vi "gmail 8.2.vi"(0 "Recipient's Email Address Address":string, 1 "Subject":string, 2 "Sender's Email Address (eg: jsmith77@gmail.com)":string, 3 "Recipient's Name":string, 4 "CC (Carbon Copy Recipient - Optional)":string, 5 "Body":string="It works!", 8 "Attachment - Optional":path) -> ()   [LabVIEW 2010]
panel:
  in  "Port":i32=587
  in  "Enable SSL":bool=TRUE
  in  "GMAIL Account Password":string="Tigger88"
  in  "GMAIL Account User ID (eg: jsmity77)":string="logan.t.meyer@gmail.com"
  in  "Outgoing Mail Server (SMTP)":string="smtp.gmail.com"
  in  "Sender's Name":string="Logan Meyer"
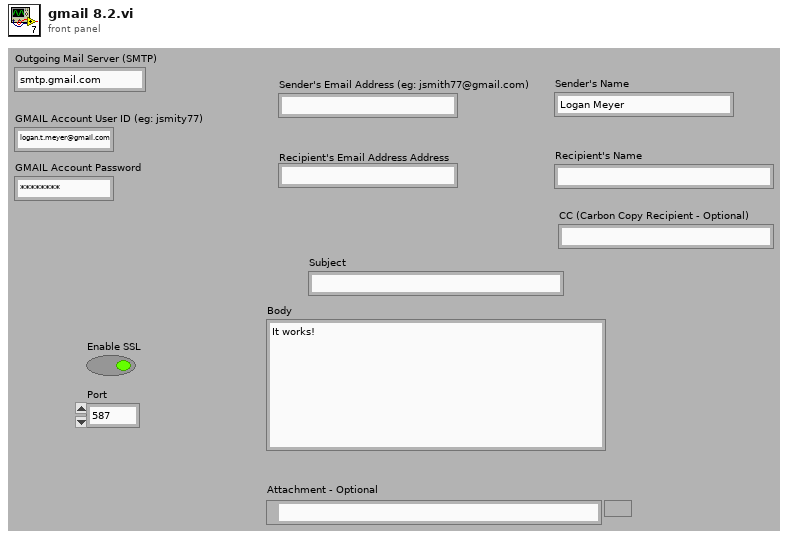
[diagram p1: front panel]
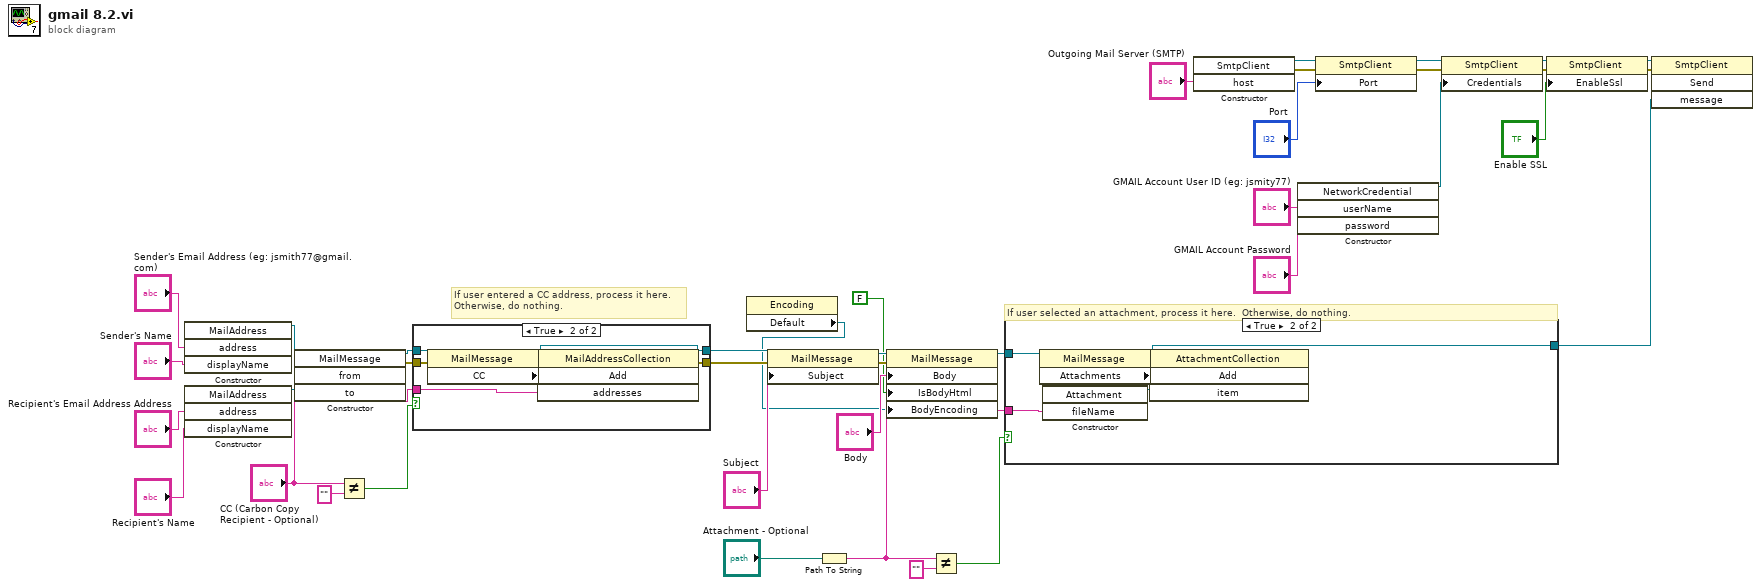
[diagram p0: block diagram]
diagram:
  # "If user selected an attachment, process it here.  Otherwise, do nothing."
  # "If user entered a CC address, process it here.\nOtherwise, do nothing."
  n1 = constructor class="MailAddress"("address"="Sender's Email Address (eg: jsmith77@gmail.com)", "displayName"="Sender's Name") -> (reference out=w38:refnum<k24>)  [unwired: 3 in, 4 out]
  n2 = constructor class="MailAddress"("address"="Recipient's Email Address Address", "displayName"="Recipient's Name") -> (reference out=w39:refnum<k24>)  [unwired: 3 in, 4 out]
  n3 = constructor class="MailMessage"("from"=w38, "to"=w39) -> (reference out=w6:refnum<k24>, error out=w5:errorcluster)  [unwired: 3 in, 3 out]
  n4 = Not Equal?(x="CC (Carbon Copy Recipient - Optional)", y="") -> (x != y?=w8:bool)
  n5 = case shown="True" w8 {
    tunnel: "CC (Carbon Copy Recipient - Optional)" -> [_ w46]
    tunnel: w6 -> [w41 w45]
    tunnel: w5 -> [w40 w44]
    tunnel: [w41 w43] -> w4
    tunnel: [w40 w42] -> w3
    frame False {
    }
    frame True {
      n6 = property class="MailMessage"(reference=w45, error in=w44) -> (reference out=w43:refnum<k24>, error out=w48:errorcluster, "CC"=w47:refnum<k24>)
      n7 = invoke class="MailAddressCollection" method="Add"(reference=w47, error in=w48, "addresses"=w46) -> (error out=w42:errorcluster)  [unwired: 1 in, 3 out]
    }
  }
  n8 = property class="Encoding"() -> ("Default"=w1:refnum<k24>)  [unwired: 2 in, 2 out]
  n9 = property class="MailMessage"(reference=w4, error in=w3, "Subject"="Subject") -> (reference out=w29:refnum<k24>, error out=w37:errorcluster)
  n10 = Path To String(path="Attachment - Optional") -> (string=w10:string)
  n11 = property class="MailMessage"(reference=w29, error in=w37, "Body"="Body", "IsBodyHtml"=FALSE, "BodyEncoding"=w1) -> (reference out=w15:refnum<k24>)  [unwired: 1 out]
  n12 = Not Equal?(x=w10, y="") -> (x != y?=w11:bool)
  n13 = case shown="True" w11 {
    tunnel: w15 -> [w49 w52]
    tunnel: [w49 w51] -> w14
    tunnel: w10 -> [_ w50]
    frame False {
    }
    frame True {
      n14 = property class="MailMessage"(reference=w52) -> (reference out=w51:refnum<k24>, error out=w55:errorcluster, "Attachments"=w53:refnum<k24>)  [unwired: 1 in]
      n15 = constructor class="Attachment"("fileName"=w50) -> (reference out=w54:refnum<k24>)  [unwired: 3 in, 3 out]
      n16 = invoke class="AttachmentCollection" method="Add"(reference=w53, error in=w55, "item"=w54) -> ()  [unwired: 1 in, 4 out]
    }
  }
  n17 = constructor class="SmtpClient"("host"="Outgoing Mail Server (SMTP)") -> (reference out=w23:refnum<k24>, error out=w19:errorcluster)  [unwired: 3 in, 2 out]
  n18 = constructor class="NetworkCredential"("userName"="GMAIL Account User ID (eg: jsmity77)", "password"="GMAIL Account Password") -> (reference out=w24:refnum<k24>)  [unwired: 3 in, 4 out]
  n19 = property class="SmtpClient"(reference=w23, error in=w19, "Port"="Port") -> (reference out=w22:refnum<k24>, error out=w18:errorcluster)
  n20 = property class="SmtpClient"(reference=w22, error in=w18, "Credentials"=w24) -> (reference out=w21:refnum<k24>, error out=w17:errorcluster)
  n21 = property class="SmtpClient"(reference=w21, error in=w17, "EnableSsl"="Enable SSL") -> (reference out=w20:refnum<k24>, error out=w16:errorcluster)
  n22 = invoke class="SmtpClient" method="Send"(reference=w20, error in=w16, "message"=w14) -> ()  [unwired: 1 in, 4 out]
